vi "Calibration - Temperature.vi"() -> ()   [LabVIEW 2016]
uses:
  calibration states.ctl
panel:
  out "Read indicator":bool
  out "Reading, C":dbl
  out "Status":string
  in  "Calibration Temperature, C":i8=100
  in  "Cancel":bool
  in  "Calibrate":bool
  # "ATLAS SCIENTIFIC\nTEMPERATURE SENSOR CALIBRATION"
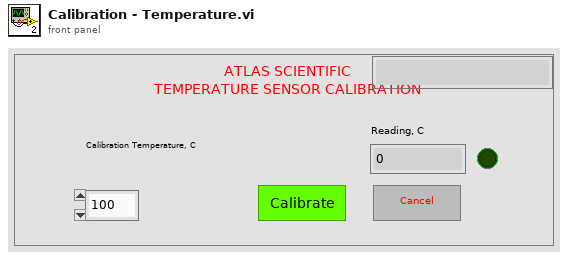
[diagram p1: front panel]
types:
  T1 = enum32{"Invalid", "Standard", "Closed", "Hidden", "Minimized", "Maximized"}
  T2 = typedef "Visa com cluster def (subVI).ctl" = cluster{"Sensor":string, "VISA resource name":refnum<visa-resource-name>, "error in/out":errorcluster, "bytes read":u32, "Com found ?":bool}
  T3 = typedef "calibration states.ctl" = string
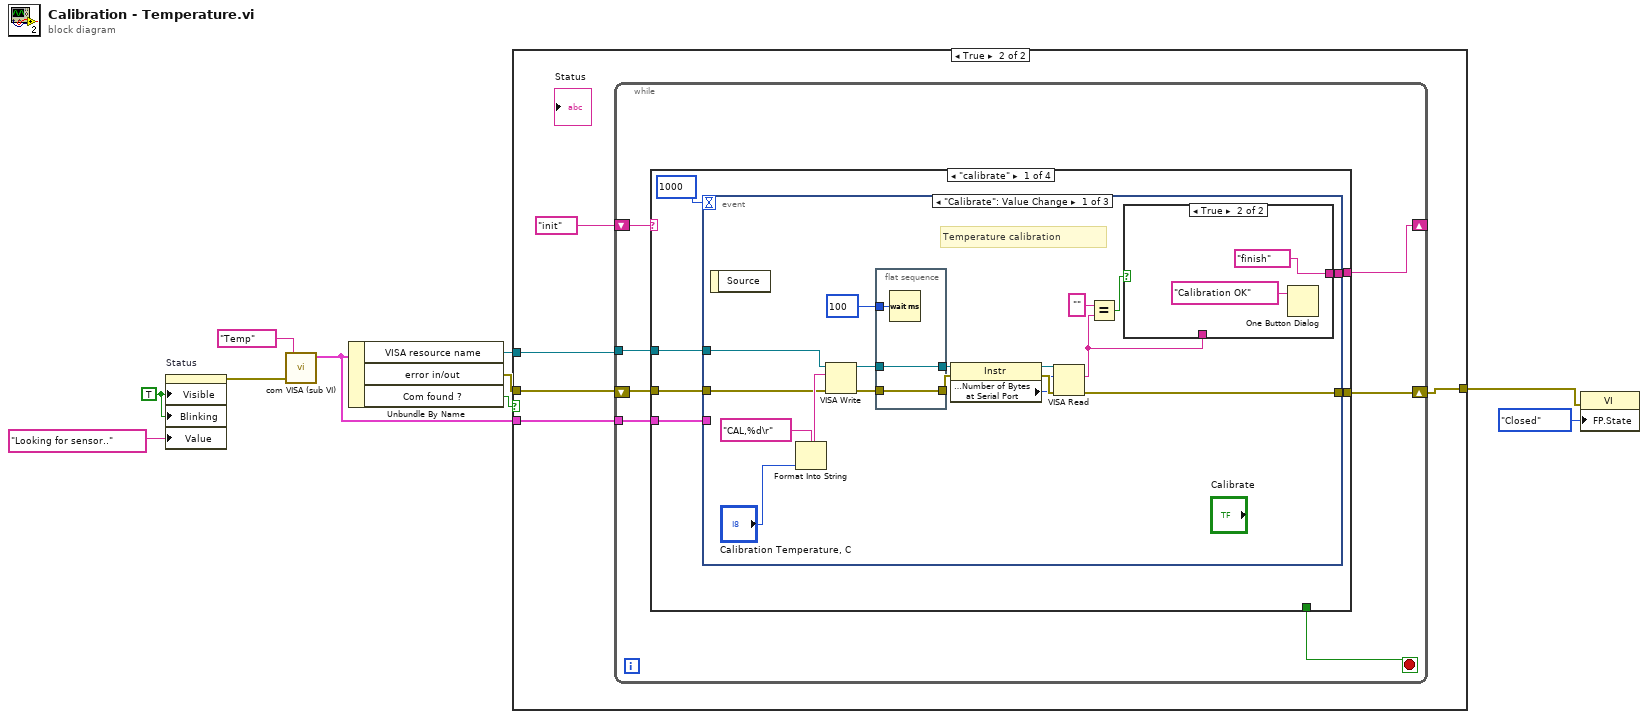
[diagram p0: block diagram]
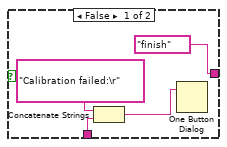
[diagram p3: hidden frame]
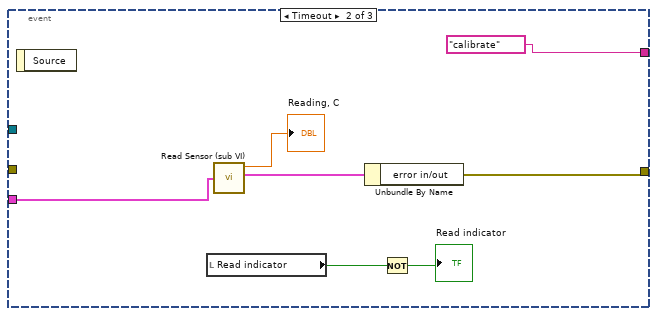
[diagram p4: hidden frame]
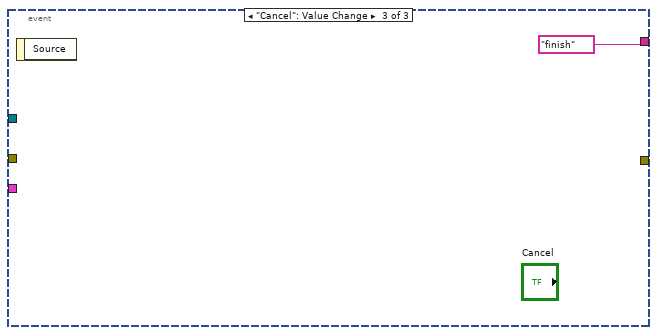
[diagram p5: hidden frame]
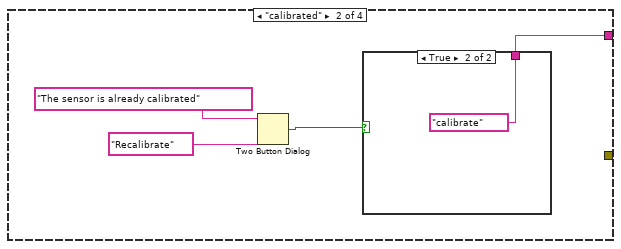
[diagram p6: hidden frame]
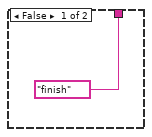
[diagram p7: hidden frame]
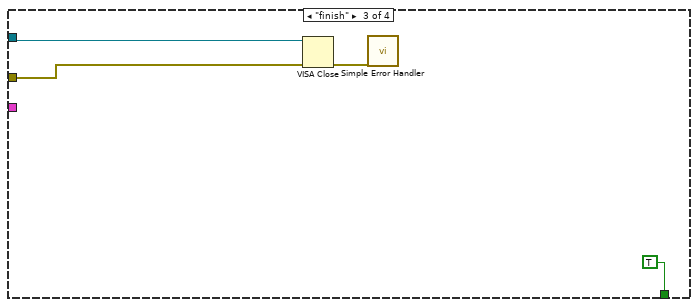
[diagram p8: hidden frame]
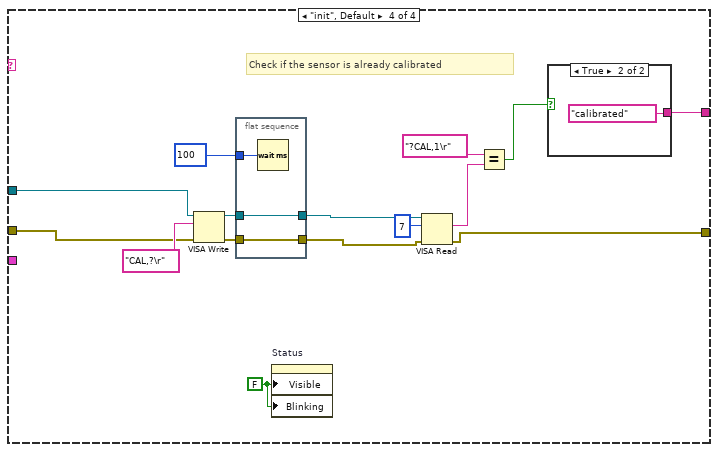
[diagram p9: hidden frame]
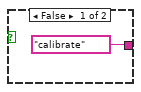
[diagram p10: hidden frame]
diagram:
  w7 = TRUE ("Visible")
  n1 = property on="Status" class="Str"("Visible"=w7, "Blinking"=w7, "Value"="Looking for sensor.." ("Status")) -> (error out=w6:errorcluster)  [unwired: 2 in, 1 out]
  n2 = call "com VISA (sub VI).vi"("Sensor"="Temp", "entrée d'erreur (pas d'erreur)"=w6) -> ("Output cluster"=w5:T2)  [unwired: 2 in, 1 out]
  n3 = Unbundle By Name(w5) -> ("VISA resource name"=w9:refnum<visa-resource-name>, "error in/out"=w8:errorcluster, "Com found ?"=w1:bool)
  n4 = case shown="True" w1 {
    tunnel: w9 -> [_ w14]
    tunnel: w8 -> [_ w13]
    tunnel: w5 -> [_ w12]
    tunnel: [_ w11] -> w2
    frame False {
    }
    frame True {
      n5 = while {
        tunnel: w14 -> [w21]
        shift-right: [w20] -> _
        shift-left: T3 "init" ("State Calibr") -> [w22]
        shift-right: [w17] -> w11
        shift-left: w13 -> [w18]
        tunnel: w12 -> [w16]
        stop <- w19 stop-if-true
        n6 = case shown="\"calibrate\"" w22 {
          tunnel: w21 -> [w28 _ w71 w80]
          tunnel: [w27 w64 _ w78] -> w20
          tunnel: [_ _ TRUE _] -> w19
          tunnel: w18 -> [w26 _ w70 w76]
          tunnel: [w25 _ _ w75] -> w17
          tunnel: w16 -> [w23 _ _ _]
          frame "calibrate" {
            n7 = event shown="[0] \"Calibrate\": Value Change" {
              selector: _ -> [_ _ _]
              dyn-events: _ -> [_ _ _]
              timeout: 1000 -> [_ _ _]
              tunnel: w28 -> [w39 _ _]
              tunnel: [w33 T3 "calibrate" ("State Calibr") T3 "finish" ("State Calibr")] -> w27
              tunnel: w26 -> [w30 _ _]
              tunnel: [w29 w57 _] -> w25
              tunnel: w23 -> [_ w56 _]
              event "Calibrate": Value Change {
                # "Temperature calibration"
                n8 = event-data() -> ()  [unwired: 1 in, 1 out]
                n9 = Format Into String(format string="CAL,%d\r", "Calibration Temperature, C") -> (resulting string=w42:string)  [unwired: 2 in, 1 out]
                n10 = VISA Write(VISA resource name=w39, write buffer=w42, error in (no error)=w30) -> (VISA resource name out=w45:refnum<visa-resource-name>, error out=w46:errorcluster)  [unwired: 1 out]
                n11 = flat-sequence {
                  tunnel: w46 -> [w48]
                  tunnel: [w48] -> w35
                  tunnel: w45 -> [w47]
                  tunnel: [w47] -> w34
                  tunnel: u32 100 ("delay before read (ms)") -> [w49]
                  frame #0 {
                    n12 = Wait (ms)(milliseconds to wait=w49) -> ()  [unwired: 1 out]
                  }
                }
                n13 = property class="Instr"(reference=w34, error in=w35) -> (reference out=w38:refnum<visa-resource-name>, error out=w37:errorcluster, "Serial Settings:Number of Bytes at Serial Port"=w36:u32)
                n14 = VISA Read(VISA resource name=w38, byte count=w36, error in (no error)=w37) -> (read buffer=w31:string, error out=w29:errorcluster)  [unwired: 2 out]
                n15 = Equal?(x="" ("Response 2"), y=w31) -> (x = y?=w32:bool)
                n16 = case shown="True" w32 {
                  tunnel: [T3 "finish" ("State Calibr") T3 "finish" ("State Calibr")] -> w33
                  tunnel: w31 -> [w52 _]
                  frame False {
                    n17 = Concatenate Strings("Calibration failed:\r" ("message"), w52) -> (w50:string)
                    n18 = One Button Dialog(message=w50) -> ()  [unwired: 1 in, 1 out]
                  }
                  frame True {
                    n19 = One Button Dialog(message="Calibration OK") -> ()  [unwired: 1 in, 1 out]
                  }
                }
              }
              event Timeout {
                n20 = event-data() -> ()  [unwired: 1 in, 1 out]
                n21 = local read "Read indicator"() -> (w61:bool)
                n22 = call "Read Sensor (sub VI).vi"("Input cluster"=w56) -> ("Reading"=→"Reading, C":dbl, "Output cluster"=w59:T2)  [unwired: 2 in]
                n23 = Unbundle By Name(w59) -> ("error in/out"=w57:errorcluster)
                n24 = Not(x=w61) -> (.not. x?=→"Read indicator":bool)
              }
              event "Cancel": Value Change {
                n25 = event-data() -> ()  [unwired: 1 in, 1 out]
              }
            }
          }
          frame "calibrated" {
            n26 = Two Button Dialog(message="The sensor is already calibrated", 2:"Recalibrate" ("T button name (\"OK\")")) -> (T button?=w65:bool)  [unwired: 1 in]
            n27 = case shown="True" w65 {
              tunnel: [T3 "finish" ("State Calibr") T3 "calibrate" ("State Calibr")] -> w64
              frame False {
              }
              frame True {
              }
            }
          }
          frame "finish" {
            n28 = VISA Close(VISA resource name=w71, error in (no error)=w70) -> (error out=w72:errorcluster)
            n29 = call <vilib>:"Simple Error Handler.vi"("error in (no error)"=w72) -> ()  [unwired: 1 in, 8 out]
          }
          frame "init", Default {
            w74 = FALSE ("Visible")
            # "Check if the sensor is already calibrated"
            n30 = VISA Write(VISA resource name=w80, write buffer="CAL,?\r", error in (no error)=w76) -> (VISA resource name out=w82:refnum<visa-resource-name>, error out=w81:errorcluster)  [unwired: 1 out]
            n31 = flat-sequence {
              tunnel: w81 -> [w92]
              tunnel: [w92] -> w86
              tunnel: w82 -> [w91]
              tunnel: [w91] -> w88
              tunnel: u32 100 ("delay before read (ms)") -> [w93]
              frame #0 {
                n32 = Wait (ms)(milliseconds to wait=w93) -> ()  [unwired: 1 out]
              }
            }
            n33 = property on="Status" class="Str"("Visible"=w74, "Blinking"=w74) -> ()  [unwired: 2 in, 2 out]
            n34 = VISA Read(VISA resource name=w88, byte count=u32 7, error in (no error)=w86) -> (read buffer=w77:string, error out=w75:errorcluster)  [unwired: 2 out]
            n35 = Equal?(x="?CAL,1\r" ("Response 2"), y=w77) -> (x = y?=w79:bool)
            n36 = case shown="True" w79 {
              tunnel: [T3 "calibrate" ("State Calibr") T3 "calibrated" ("State Calibr")] -> w78
              frame False {
              }
              frame True {
              }
            }
          }
        }
      }
    }
  }
  n37 = property class="VI"(error in=w2, "FP.State"=T1."Closed" ("Front Panel Window:State")) -> ()  [unwired: 1 in, 2 out]
